vi "send response.vi"(6 "udp message":string, 7 "connection ID out":refnum<k16>, 8 "error in (no error)":errorcluster, 9 "port":u16, 10 "address":u32, 11 "Send Notification in":refnum<class "Send Notification.lvclass">) -> (0 "error out":errorcluster, 3 "Send Notification out":refnum<class "Send Notification.lvclass">)   [LabVIEW 2025, in "Send Notification.lvclass"]
uses:
  Send Notification.lvclass
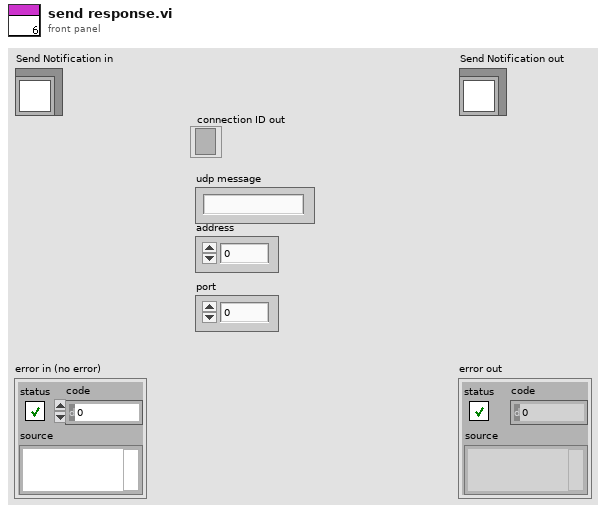
[diagram p1: front panel]
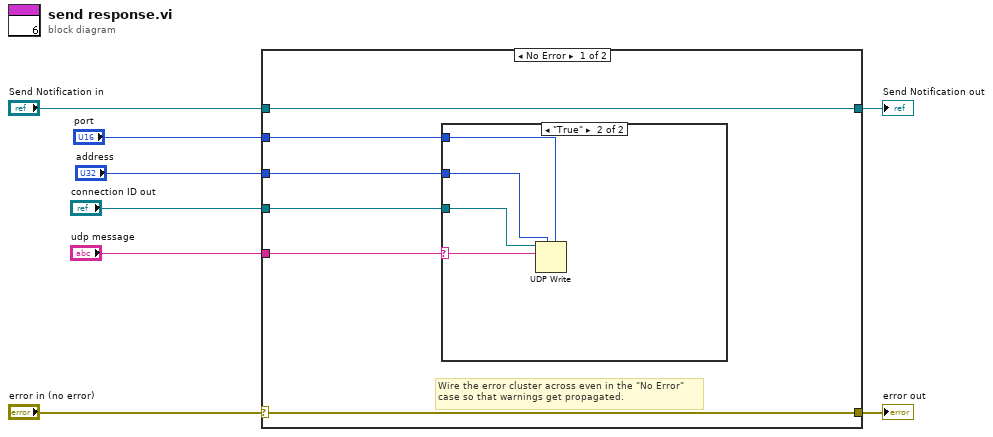
[diagram p0: block diagram]
diagram:
  n1 = case shown="No Error" "error in (no error)" {
    selector: "error in (no error)" -> [w13 w20]
    tunnel: [w13 w20] -> w7
    tunnel: [w14 w19] -> w5
    tunnel: "Send Notification in" -> [w14 w19]
    tunnel: "connection ID out" -> [w11 _]
    tunnel: "udp message" -> [w12 _]
    tunnel: "address" -> [w10 _]
    tunnel: "port" -> [w9 _]
    frame No Error {
      # "Wire the error cluster across even in the \"No Error\"\ncase so that warnings get propagated."
      n2 = case shown="\"True\"" w12 {
        selector: w12 -> [_ w18]
        tunnel: w11 -> [_ w17]
        tunnel: w10 -> [_ w16]
        tunnel: w9 -> [_ w15]
        frame "False", Default {
        }
        frame "True" {
          n3 = UDP Write(address=w16, port or service name=w15, connection ID=w17, data in=w18) -> ()  [unwired: 2 in, 2 out]
        }
      }
    }
    frame Error {
    }
  }
  "error out" <- w7
  "Send Notification out" <- w5
